vi "AuMT8852B Tester Hardware Information.vi"(8 "error in (no error)":errorcluster, 11 "VISA session":refnum<visa-resource-name>) -> (0 "error out":errorcluster, 2 "error code":i32, 3 "VISA session out":refnum<visa-resource-name>, 4 "Hardware Information":T1)   [LabVIEW 2017]
doc: "Anritsu MT8852B Bluetooth Tester\n\nObtains the RF PCB serial number and revision and the Control PCB serial number and revision of the tester."
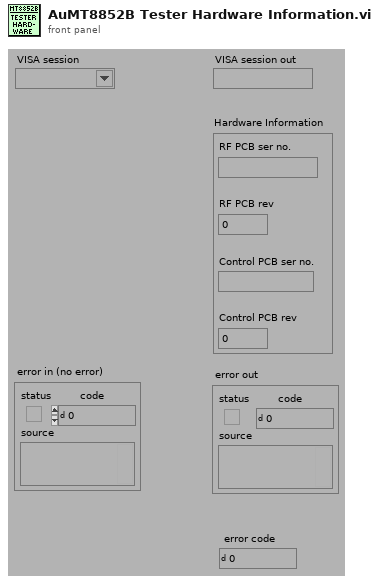
[diagram p1: front panel]
types:
  T1 = cluster{"RF PCB ser no.":string, "RF PCB rev":i32, "Control PCB ser no.":string, "Control PCB rev":i32}
  T2 = enum16{"Simulate", "Range check", "Cache", "Query instrument status"}
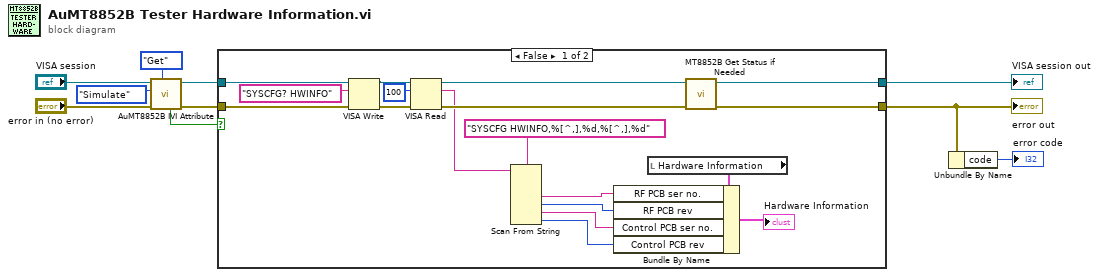
[diagram p0: block diagram]
diagram:
  n1 = call <instrlib>:"AuMT8852B IVI Attribute.vi"("Set/Get (Set)"=enum16{"Set", "Get"}."Get", "error in (no error)"="error in (no error)", "Flag (Simulate)"=T2."Simulate", "VISA session"="VISA session") -> ("error out"=w7:errorcluster, "VISA session out"=w9:refnum<visa-resource-name>, "Value out"=w3:bool)  [unwired: 5 in]
  n2 = case shown="False" w3 {
    tunnel: [w20 w30] -> w10
    tunnel: [w19 w29] -> w1
    tunnel: w9 -> [w27 w30]
    tunnel: w7 -> [w26 w29]
    frame False {
      n3 = VISA Write(VISA resource name=w27, write buffer="SYSCFG? HWINFO" ("write buffer (\"\")"), error in (no error)=w26) -> (VISA resource name out=w25:refnum<visa-resource-name>, error out=w24:errorcluster)  [unwired: 1 out]
      n4 = VISA Read(VISA resource name=w25, byte count=u32 100 ("byte count (0)"), error in (no error)=w24) -> (VISA resource name out=w17:refnum<visa-resource-name>, read buffer=w15:string, error out=w18:errorcluster)  [unwired: 1 out]
      n5 = Scan From String(format string="SYSCFG HWINFO,%[^,],%d,%[^,],%d" ("write buffer (\"\")"), input string=w15) -> (output 1=w14:string, output 2=w11:i32, output 3=w13:string, output 4=w12:i32)  [unwired: 6 in, 3 out]
      n6 = local read "Hardware Information"() -> (w22:T1)
      n7 = Bundle By Name(cluster=w22, "RF PCB ser no."=w14, "RF PCB rev"=w11, "Control PCB ser no."=w13, "Control PCB rev"=w12) -> (→"Hardware Information":T1)
      n8 = call <instrlib>:"MT8852B Get Status if Needed.vi"("error in (no error)"=w18, "VISA session"=w17) -> ("error out"=w19:errorcluster, "VISA session out"=w20:refnum<visa-resource-name>)  [unwired: 8 in]
    }
    frame True {
    }
  }
  "error out" <- w1
  "VISA session out" <- w10
  n9 = Unbundle By Name(w1) -> ("code"=→"error code":i32)
